vi "valuePathSearch.vi"(8 "error in (no error)":errorcluster, 10 "Array":string[](array[string]), 11 "ConsoleViewer in":refnum<class "ConsoleViewer.lvclass">) -> (0 "error out":errorcluster, 2 "Array 2":string[][](array[string]), 3 "ConsoleViewer out":refnum<class "ConsoleViewer.lvclass">)   [LabVIEW 2009, in "Views.lvlib" / "ConsoleViewer.lvclass"]
uses:
  ConsoleViewer.lvclass
  ConsoleViewer.lvclass/ConsoleViewer.ctl
  Tools/CommandProcessor/CommandEvents/CommandEvents.lvclass
  Tools/SettingsEventManager/SettingsEventsManager.lvclass
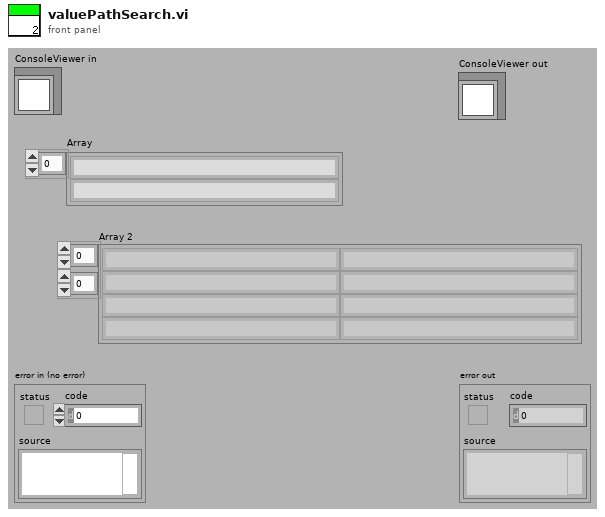
[diagram p1: front panel]
types:
  T1 = cluster{"settingsFrontEndEvents":cluster{"loadSettingsFromPath":refnum<user-event>, "lookUpElementEvent":refnum<user-event>, "saveSettings":refnum<user-event>, "loadSettings":refnum<user-event>, "close":refnum<user-event>, "replaceElement":refnum<user-event>, "findParentNodes":refnum<user-event>, "createNode":refnum<user-event>}, "settingBackEndEvents":cluster{"defaultSettingsPathRequest":refnum<user-event>, "searchResultEvent":refnum<user-event>, "settingsSaved":refnum<user-event>, "settingsLoaded":refnum<user-event>, "foundParentNode":refnum<user-event>}}
  T2 = cluster{"newCommand":refnum<user-event>, "textUpdate":refnum<user-event>}
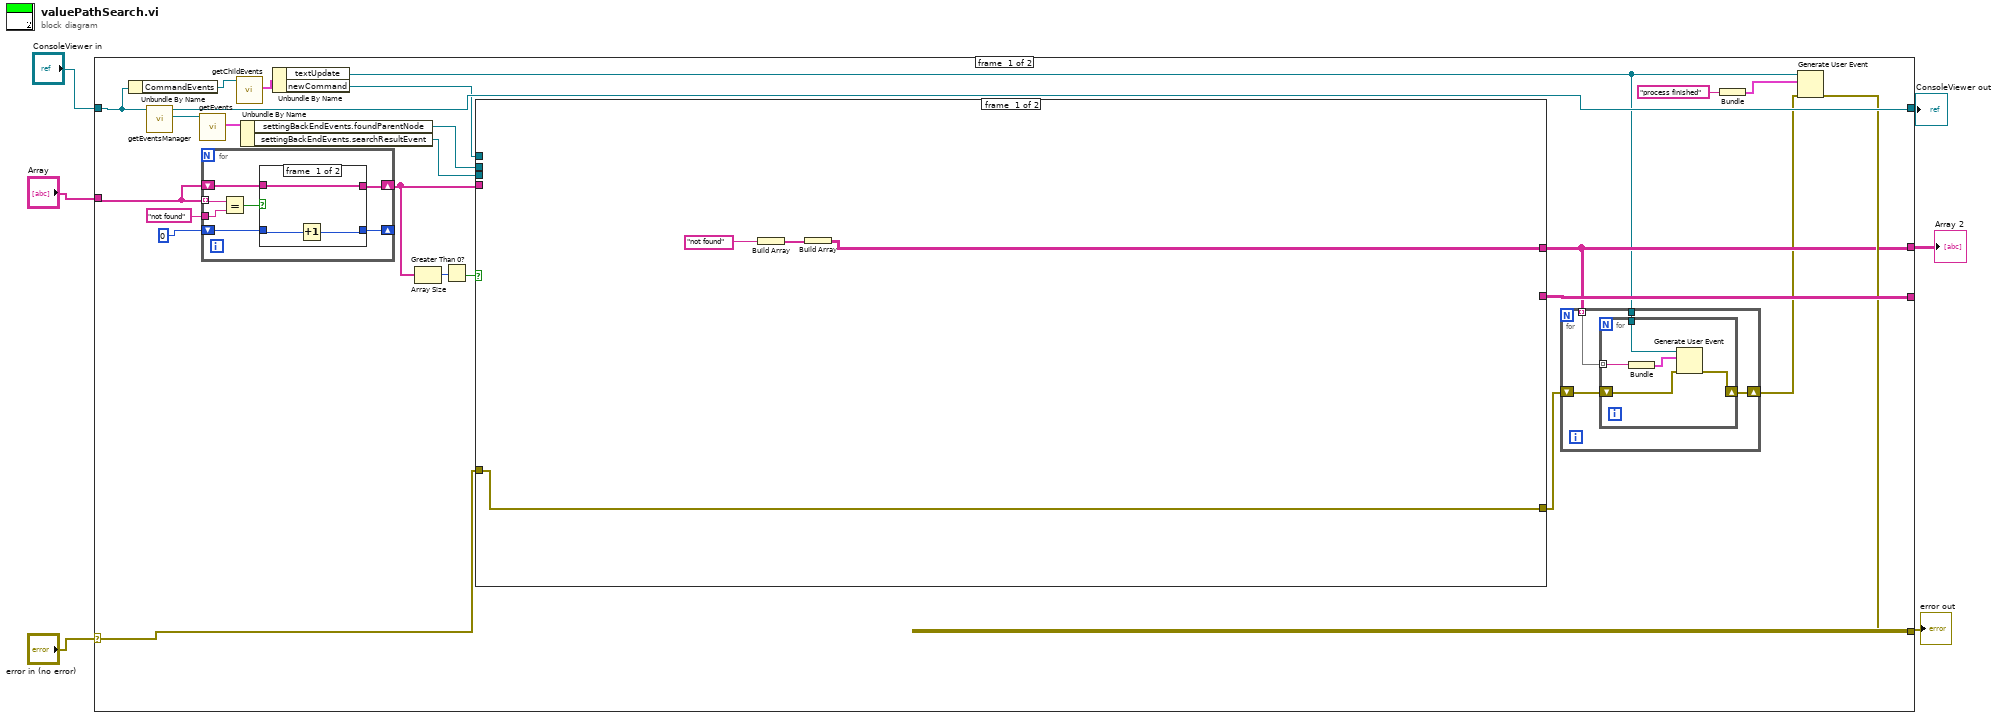
[diagram p0: block diagram]
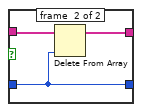
[diagram p2: hidden frame]
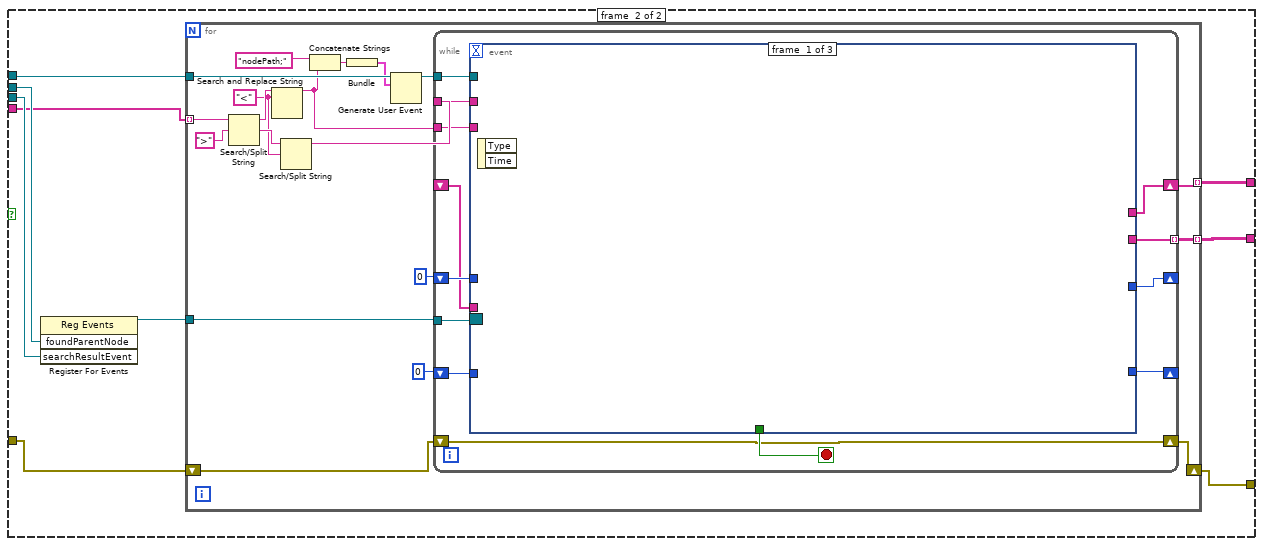
[diagram p3: hidden frame]
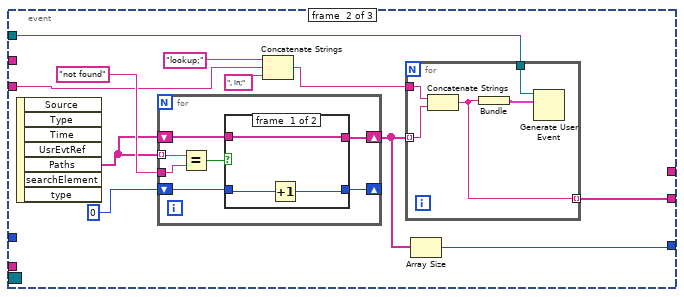
[diagram p4: hidden frame]
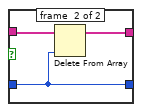
[diagram p5: hidden frame]
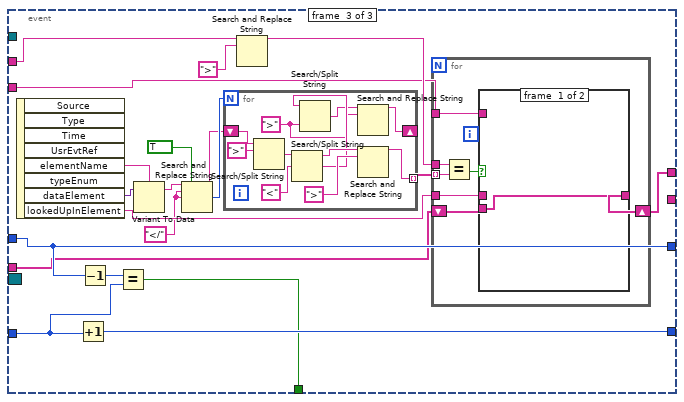
[diagram p6: hidden frame]
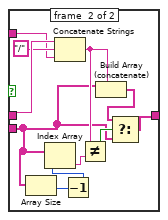
[diagram p7: hidden frame]
diagram:
  n1 = case shown="No Error" "error in (no error)" {
    selector: "error in (no error)" -> [w12 w178]
    tunnel: [w11 w178] -> w5
    tunnel: [w25 w177] -> w3
    tunnel: "ConsoleViewer in" -> [w23 w177]
    tunnel: "Array" -> [w29 _]
    tunnel: [w10 _] -> w1
    tunnel: [w15 _] -> _
    frame #0 {
      n2 = Unbundle By Name(w23) -> ("CommandEvents"=w22:refnum<class "CommandEvents.lvclass">)
      n3 = call-dynamic "getEventsManager.vi"("SettingsViewer.lvclass in"=w23) -> ("Tools.lvlib:Settings.lvlib:SettingsEventsManager.lvclass"=w24:refnum<class "SettingsEventsManager.lvclass">, "SettingsViewer.lvclass out"=w25:refnum<class "ConsoleViewer.lvclass">)  [unwired: 8 in, 1 out]
      n4 = call-dynamic "getEvents.vi"("SettingsEventsManager in"=w24) -> ("settingsEvents"=w19:T1)  [unwired: 8 in, 2 out]
      n5 = for {
        tunnel: w29 -> [w45] mode=indexing
        tunnel: "not found" -> [w46]
        shift-right: [w43] -> _
        shift-left: 0 -> [w42]
        shift-right: [w41] -> w16
        shift-left: w29 -> [w44]
        n6 = Equal?(x=w45, y=w46) -> (x = y?=w40:bool)
        n7 = case shown="False" w40 {
          tunnel: w44 -> [w47 w51]
          tunnel: w42 -> [w49 w52]
          tunnel: [w48 w52] -> w43
          tunnel: [w47 w50] -> w41
          frame #0 {
            n8 = Increment(x=w49) -> (x+1=w48:i32)
          }
          frame #1 {
            n9 = Delete From Array(array=w51, index=w52) -> (array with subset deleted=w50:string[])  [unwired: 1 in, 1 out]
          }
        }
      }
      n10 = call-dynamic "getChildEvents.vi"("CommandEvents in"=w22) -> ("Events"=w21:T2)  [unwired: 8 in, 2 out]
      n11 = Unbundle By Name(w19) -> ("settingBackEndEvents.foundParentNode"=w18:refnum<user-event>, "settingBackEndEvents.searchResultEvent"=w17:refnum<user-event>)
      n12 = Unbundle By Name(w21) -> ("textUpdate"=w8:refnum<user-event>, "newCommand"=w20:refnum<user-event>)
      n13 = Array Size(array=w16) -> (size(s)=w27:i32)
      n14 = Greater Than 0?(x=w27) -> (x > 0?=w26:bool)
      n15 = case shown="False" w26 {
        tunnel: [w53 w60] -> w10
        tunnel: w16 -> [_ w57]
        tunnel: w20 -> [_ w62]
        tunnel: w18 -> [_ w65]
        tunnel: w17 -> [_ w63]
        tunnel: [_ w61] -> w15
        tunnel: [w55 w59] -> w9
        tunnel: w12 -> [w55 w58]
        frame #0 {
          n16 = Build Array("not found") -> (w54:string[])
          n17 = Build Array(w54) -> (w53:string[][])
        }
        frame #1 {
          n18 = register-events(w65, w63) -> (reference out=w64:refnum<event-registration>)  [unwired: 2 in, 1 out]
          n19 = for {
            tunnel: w64 -> [w84]
            tunnel: w62 -> [w80]
            tunnel: [w73] -> w61 mode=indexing
            tunnel: [w69] -> w60 mode=indexing
            tunnel: w57 -> [w66] mode=indexing
            shift-right: [w68] -> w59
            shift-left: w58 -> [w67]
            w75 = "<"
            n20 = Search/Split String(string=w66, search string/char (-)=">") -> (substring before match=w82:string, match + rest of string=w76:string)  [unwired: 1 in, 1 out]
            n21 = Search and Replace String(input string=w82, search string=w75) -> (result string=w72:string)  [unwired: 6 in, 3 out]
            n22 = Search/Split String(string=w76, search string/char (-)=w75) -> (substring before match=w71:string)  [unwired: 1 in, 2 out]
            n23 = Concatenate Strings("nodePath;", w72) -> (w79:string)
            n24 = Bundle(w79) -> (w78:cluster{string})  [unwired: 1 in]
            n25 = Generate User Event(user event=w80, event data cluster=w78) -> (user event out=w74:refnum<user-event>)  [unwired: 1 in, 1 out]
            n26 = while {
              tunnel: w84 -> [w97]
              shift-right: [w96] -> _
              shift-left: 0 -> [w91]
              tunnel: w72 -> [w95]
              tunnel: w74 -> [w94]
              tunnel: [w93] -> w73 mode=indexing
              tunnel: w71 -> [w88]
              shift-right: [w89] -> _
              shift-left: 0 -> [w90]
              shift-right: [w87] -> w69
              shift-left: _ -> [w86]
              shift-right: [w85] -> w68
              shift-left: w67 -> [w85]
              stop <- w92 stop-if-true
              n27 = event shown="[2] <searchResultEvent>: User Event" {
                selector: w97 -> [_ _ _]
                dyn-events: _ -> [_ _ _]
                timeout: _ -> [_ _ _]
                tunnel: [_ w108 w143] -> w96
                tunnel: w95 -> [_ w102 w128]
                tunnel: w94 -> [_ w99 _]
                tunnel: [_ w98 _] -> w93
                tunnel: [_ _ w144] -> w92
                tunnel: w91 -> [_ _ w143]
                tunnel: w90 -> [_ _ w145]
                tunnel: [_ _ w146] -> w89
                tunnel: w88 -> [_ _ w136]
                tunnel: [_ _ w138] -> w87
                tunnel: w86 -> [_ _ w137]
                event #0 {
                  n28 = event-data() -> ()  [unwired: 1 in, 2 out]
                }
                event #1 {
                  n29 = event-data() -> ("Paths"=w105:string[])  [unwired: 1 in, 6 out]
                  n30 = for {
                    tunnel: w105 -> [w119] mode=indexing
                    tunnel: "not found" -> [w120]
                    shift-right: [w117] -> _
                    shift-left: 0 -> [w116]
                    shift-right: [w115] -> w104
                    shift-left: w105 -> [w118]
                    n31 = Equal?(x=w119, y=w120) -> (x = y?=w114:bool)
                    n32 = case shown="False" w114 {
                      tunnel: w118 -> [w121 w125]
                      tunnel: w116 -> [w123 w126]
                      tunnel: [w122 w126] -> w117
                      tunnel: [w121 w124] -> w115
                      frame #0 {
                        n33 = Increment(x=w123) -> (x+1=w122:i32)
                      }
                      frame #1 {
                        n34 = Delete From Array(array=w125, index=w126) -> (array with subset deleted=w124:string[])  [unwired: 1 in, 1 out]
                      }
                    }
                  }
                  n35 = Concatenate Strings("lookup;", w102, ", in;") -> (w100:string)
                  n36 = for {
                    tunnel: w104 -> [w112] mode=indexing
                    tunnel: w100 -> [w113]
                    tunnel: w99 -> [w110]
                    tunnel: [w109] -> w98 mode=indexing
                    n37 = Concatenate Strings(w113, w112) -> (w109:string)
                    n38 = Bundle(w109) -> (w111:cluster{string})  [unwired: 1 in]
                    n39 = Generate User Event(user event=w110, event data cluster=w111) -> ()  [unwired: 1 in, 2 out]
                  }
                  n40 = Array Size(array=w104) -> (size(s)=w108:i32)
                }
                event #2 {
                  w130 = "</"
                  n41 = event-data() -> ("elementName"=w140:string, "dataElement"=w141:variant, "lookedUpInElement"=w139:string)  [unwired: 1 in, 5 out]
                  n42 = Increment(x=w145) -> (x+1=w146:i32)
                  n43 = Decrement(x=w143) -> (x-1=w142:i32)
                  n44 = Equal?(x=w142, y=w145) -> (x = y?=w144:bool)
                  n45 = Variant To Data(Variant=w141, type=w140) -> (data=w131:string)  [unwired: 1 in, 1 out]
                  n46 = Search and Replace String(replace all?=TRUE, input string=w131, search string=w130, replace string=w130) -> (result string=w127:string, number of replacements=w133:i32)  [unwired: 4 in, 2 out]
                  n47 = for {
                    N: w133 -> [_]
                    tunnel: [w173] -> w134 mode=indexing
                    shift-right: [w166] -> _
                    shift-left: w127 -> [w170]
                    w167 = ">"
                    n48 = Search/Split String(string=w170, search string/char (-)=">") -> (match + rest of string=w175:string)  [unwired: 1 in, 2 out]
                    n49 = Search/Split String(string=w175, search string/char (-)="<") -> (substring before match=w176:string, match + rest of string=w169:string)  [unwired: 1 in, 1 out]
                    n50 = Search/Split String(string=w169, search string/char (-)=w167) -> (match + rest of string=w168:string)  [unwired: 1 in, 2 out]
                    n51 = Search and Replace String(input string=w168, search string=w167) -> (result string=w166:string)  [unwired: 6 in, 3 out]
                    n52 = Search and Replace String(input string=w176, search string=">") -> (result string=w173:string)  [unwired: 6 in, 3 out]
                  }
                  n53 = Search and Replace String(input string=w136, search string=">") -> (result string=w132:string)  [unwired: 6 in, 3 out]
                  n54 = for {
                    tunnel: w139 -> [w153]
                    tunnel: w128 -> [w150]
                    tunnel: w134 -> [w149] mode=indexing
                    tunnel: w132 -> [w148]
                    shift-right: [w152] -> w138
                    shift-left: w137 -> [w151]
                    n55 = Equal?(x=w148, y=w149) -> (x = y?=w147:bool)
                    n56 = case shown="False" w147 {
                      tunnel: w153 -> [_ w165]
                      tunnel: [w154 w156] -> w152
                      tunnel: w151 -> [w154 w155]
                      tunnel: w150 -> [_ w163]
                      frame #0 {
                      }
                      frame #1 {
                        n57 = Array Size(array=w155) -> (size(s)=w162:i32)
                        n58 = Concatenate Strings(w165, "/", w163) -> (w158:string)
                        n59 = Decrement(x=w162) -> (x-1=w161:i32)
                        n60 = Index Array(array=w155, index=w161) -> (element=w159:string)
                        n61 = Not Equal?(x=w158, y=w159) -> (x != y?=w160:bool)
                        n62 = Build Array (concatenate)(w155, w158) -> (w157:string[])
                        n63 = Select(t=w157, s=w160, f=w155) -> (s? t:f=w156:string[])
                      }
                    }
                  }
                }
              }
            }
          }
        }
      }
      n64 = for {
        tunnel: w10 -> [w34] mode=indexing
        tunnel: w8 -> [w32]
        shift-right: [w31] -> w7
        shift-left: w9 -> [w33]
        n65 = for {
          tunnel: w34 -> [w36] mode=indexing
          tunnel: w32 -> [w38]
          shift-right: [w37] -> w31
          shift-left: w33 -> [w39]
          n66 = Bundle(w36) -> (w35:cluster{string})  [unwired: 1 in]
          n67 = Generate User Event(user event=w38, event data cluster=w35, error in=w39) -> (error out=w37:errorcluster)  [unwired: 1 out]
        }
      }
      n68 = Bundle("process finished") -> (w14:cluster{string})  [unwired: 1 in]
      n69 = Generate User Event(user event=w8, event data cluster=w14, error in=w7) -> (error out=w11:errorcluster)  [unwired: 1 out]
    }
    frame #1 {
    }
  }
  "error out" <- w5
  "ConsoleViewer out" <- w3
  "Array 2" <- w1
